vi "Compile Connection.vi"(8 "error in (no error)":errorcluster, 10 "Connection":T1, 11 "Communication Configuration":T2) -> (0 "error out":errorcluster, 3 "Compiled Connection":T3)   [LabVIEW 2017, in "Routing and Faulting System Explorer.lvlib"]
uses:
  Routing and Faulting System Explorer.lvlib
  Shared/Compiled Connection.ctl
  Shared/Communication Configuration.ctl
  Shared/Connection.ctl
  Shared/Routing and Faulting Shared.lvlib
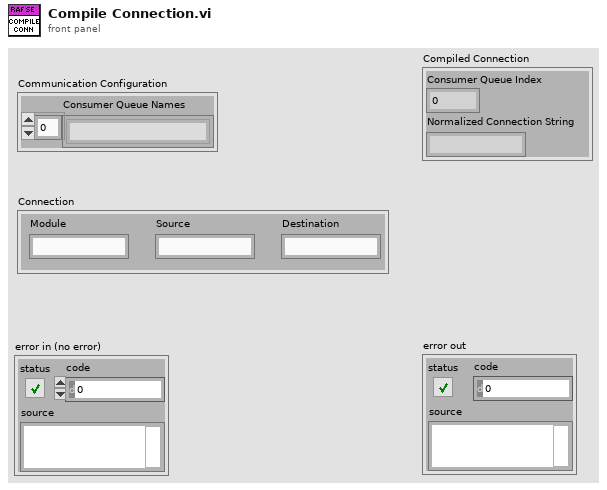
[diagram p1: front panel]
types:
  T1 = typedef "Routing and Faulting Shared.lvlib/Connection.ctl" = cluster{"Module":string, "Source":string, "Destination":string}
  T2 = typedef "Routing and Faulting Shared.lvlib/Communication Configuration.ctl" = cluster{"Consumer Queue Names":string[]}
  T3 = typedef "Routing and Faulting Shared.lvlib/Compiled Connection.ctl" = cluster{"Consumer Queue Index":i32, "Normalized Connection String":string}
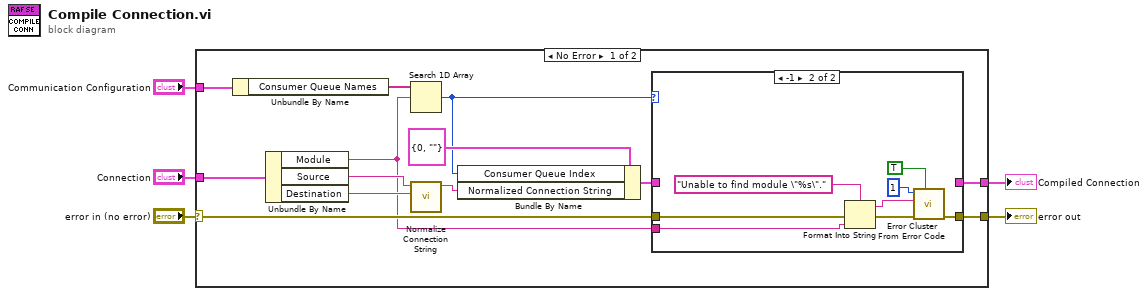
[diagram p0: block diagram]
diagram:
  n1 = case shown="No Error" "error in (no error)" {
    selector: "error in (no error)" -> [w11 w29]
    tunnel: [w7 _] -> w1
    tunnel: "Communication Configuration" -> [w13 _]
    tunnel: "Connection" -> [w12 _]
    tunnel: [w10 w29] -> w2
    frame No Error {
      n2 = Unbundle By Name(w13) -> ("Consumer Queue Names"=w14:string[])
      n3 = Unbundle By Name(w12) -> ("Module"=w6:string, "Source"=w16:string, "Destination"=w17:string)
      n4 = Search 1D Array(1D array=w14, element=w6) -> (index of element=w9:i32)  [unwired: 1 in]
      n5 = call "Normalize Connection String.vi"("Destination"=w17, "Source"=w16) -> ("Normalized Connection String"=w18:string)  [unwired: 9 in]
      n6 = Bundle By Name(cluster=T3 {"Consumer Queue Index"=0, "Normalized Connection String"=""} ("Compiled Connection"), "Consumer Queue Index"=w9, "Normalized Connection String"=w18) -> (w8:T3)
      n7 = case shown="-1" w9 {
        tunnel: [w20 w28] -> w10
        tunnel: w11 -> [w20 w24]
        tunnel: [w19 _] -> w7
        tunnel: w8 -> [w19 _]
        tunnel: w6 -> [_ w22]
        frame Default {
        }
        frame -1 {
          n8 = Format Into String(format string="Unable to find module \"%s\".", error in=w24, w22) -> (resulting string=w25:string, error out=w23:errorcluster)  [unwired: 1 in]
          n9 = call <vilib>:"Error Cluster From Error Code.vi"("show call chain? (False)"=TRUE, "error in (no error)"=w23, "error message (\"\")"=w25, "error code (0)"=1) -> ("error out"=w28:errorcluster)  [unwired: 5 in]
        }
      }
    }
    frame Error {
    }
  }
  "Compiled Connection" <- w1
  "error out" <- w2
